vi "Init Lang Box.vi"(8 "error in (no error)":errorcluster, 10 "Initial Value":string="en", 11 "ComboBox Ref in":refnum<vi>) -> (0 "error out":errorcluster, 3 "ComboBox Ref out":refnum<vi>)   [LabVIEW 2013, in "SET Project Editor.lvlib"]
uses:
  SET Project Editor.lvlib
  SET Project Data/SET Project Data.lvlib
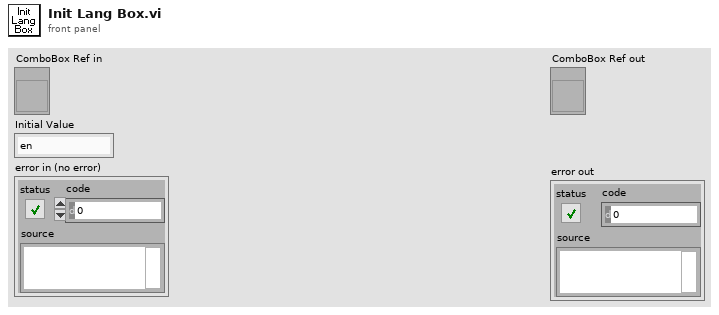
[diagram p1: front panel]
types:
  T1 = cluster{"Name":string, "Tag":string, "Code Page":u16}[]
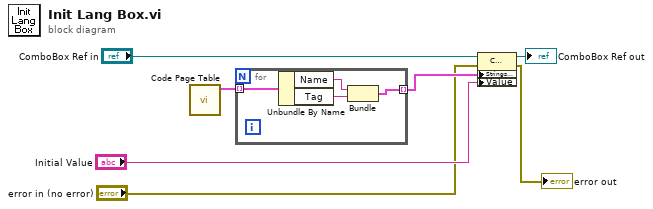
[diagram p0: block diagram]
diagram:
  n1 = call "Code Page Table.vi"() -> ("Code Page Table"=w7:T1)  [unwired: 11 in]
  n2 = for {
    tunnel: w7 -> [w11] mode=indexing
    tunnel: [w8] -> w5 mode=indexing
    n3 = Unbundle By Name(w11) -> ("Name"=w10:string, "Tag"=w9:string)
    n4 = Bundle("Name"=w10, "Tag"=w9) -> (w8:cluster{"Name":string, "Tag":string})  [unwired: 1 in]
  }
  n5 = property class="CmbBox"(reference="ComboBox Ref in", error in="error in (no error)", "Strings And Values[]"=w5, "Value"="Initial Value") -> (reference out=→"ComboBox Ref out":refnum<vi>, error out=→"error out":errorcluster)
